vi "Add Tree Location.vi"(5 "Property Name":string, 7 "Property Value":string, 8 "error in (no error)":errorcluster, 9 "Tree Items Created In":variant, 10 "Tree Parent Tag In":string, 11 "TreeControl in":refnum<vi>) -> (0 "error out":errorcluster, 1 "Tree Items Created Out":variant, 2 "Tree Parent Tag Out":string)   [LabVIEW 2017, in "XTree.xctl"]
doc: "Adds a single tree location, if it does not already exist in the Tree Items Created variant."
uses:
  <vilib>/addons/_NIFileIO/XTree/XTree.xctl
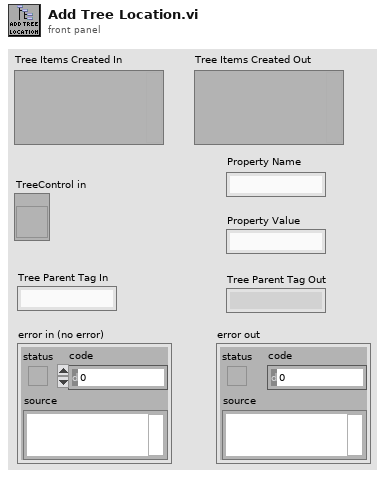
[diagram p1: front panel]
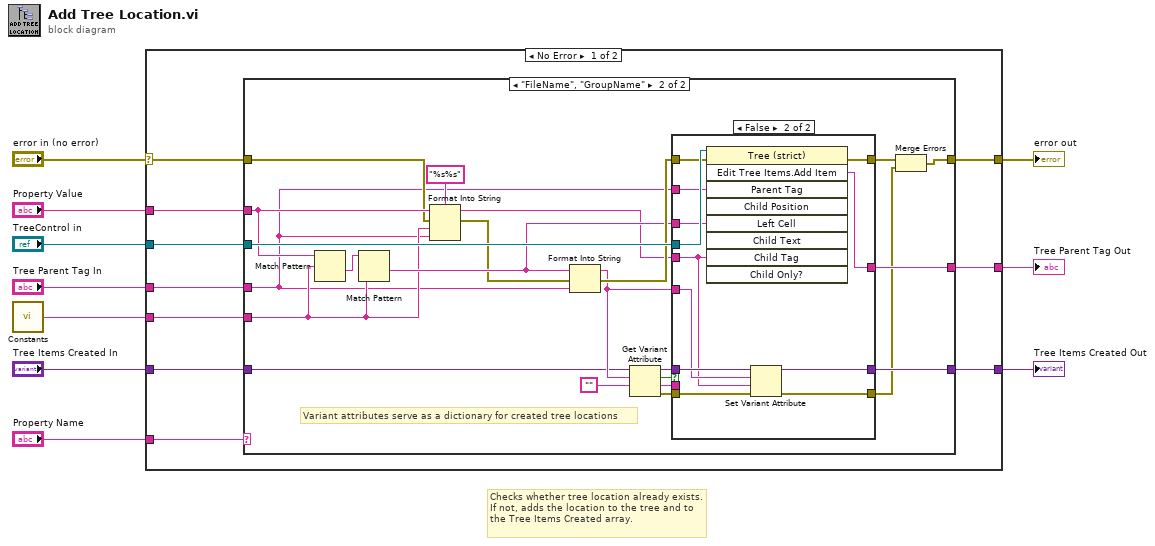
[diagram p0: block diagram]
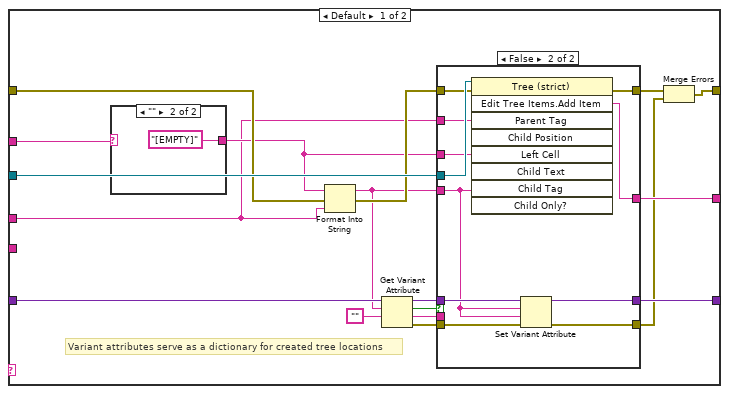
[diagram p2: hidden frame]
diagram:
  # "Checks whether tree location already exists. If not, adds the location to the tree and to the Tree Items Created array."
  n1 = call <vilib>:"Constants.vi"() -> ("String Delimeter"=w4:string)  [unwired: 5 in]
  n2 = case shown="No Error" "error in (no error)" {
    selector: "error in (no error)" -> [w17 w96]
    tunnel: "Tree Parent Tag In" -> [w15 w97]
    tunnel: [w20 w96] -> w9
    tunnel: [w19 w97] -> w8
    tunnel: "TreeControl in" -> [w18 _]
    tunnel: "Property Value" -> [w16 _]
    tunnel: w4 -> [w14 _]
    tunnel: "Property Name" -> [w13 _]
    tunnel: "Tree Items Created In" -> [w12 w95]
    tunnel: [w11 w95] -> w1
    frame No Error {
      n3 = case shown="\"FileName\", \"GroupName\"" w13 {
        tunnel: [w24 w58] -> w20
        tunnel: [w38 w78] -> w19
        tunnel: w18 -> [w37 w77]
        tunnel: w17 -> [w36 w72]
        tunnel: w16 -> [w35 w73]
        tunnel: w15 -> [w32 w67]
        tunnel: w14 -> [_ w70]
        tunnel: w12 -> [w31 w65]
        tunnel: [w26 w61] -> w11
        frame Default {
          # "Variant attributes serve as a dictionary for created tree locations"
          n4 = case shown="\"\"" w35 {
            selector: w35 -> [w39 _]
            tunnel: [w39 "[EMPTY]"] -> w33
            frame Default {
            }
            frame "" {
            }
          }
          n5 = Format Into String(initial string=w33, error in=w36, w32) -> (resulting string=w30:string, error out=w34:errorcluster)  [unwired: 1 in]
          n6 = Get Variant Attribute(Variant=w31, name=w30, default value (empty Variant)="") -> (duplicate Variant=w28:variant, found=w29:bool, value=w25:string, error out=w27:errorcluster)  [unwired: 1 in]
          n7 = case shown="False" w29 {
            tunnel: w37 -> [_ w55]
            tunnel: w34 -> [w44 w54]
            tunnel: [w43 w53] -> w38
            tunnel: [w44 w52] -> w23
            tunnel: w32 -> [_ w51]
            tunnel: w33 -> [_ w50]
            tunnel: w30 -> [_ w48]
            tunnel: w28 -> [w42 w49]
            tunnel: w27 -> [w41 w47]
            tunnel: [w42 w46] -> w26
            tunnel: w25 -> [w43 _]
            tunnel: [w41 w45] -> w22
            frame True {
            }
            frame False {
              n8 = invoke class="Tree (strict)" method="Edit Tree Items.Add Item"(reference=w55, error in=w54, "Parent Tag"=w51, "Left Cell"=w50, "Child Tag"=w48) -> (error out=w52:errorcluster, "Edit Tree Items:Add Item"=w53:string)  [unwired: 4 in, 7 out]
              n9 = Set Variant Attribute(Variant=w49, name=w48, value=w48, error in=w47) -> (Variant out=w46:variant, error out=w45:errorcluster)  [unwired: 1 out]
            }
          }
          n10 = Merge Errors(w23, w22) -> (w24:errorcluster)
        }
        frame "FileName", "GroupName" {
          # "Variant attributes serve as a dictionary for created tree locations"
          n11 = Match Pattern(string=w73, regular expression=w70) -> (after substring=w75:string)  [unwired: 1 in, 3 out]
          n12 = Match Pattern(string=w75, regular expression=w70) -> (after substring=w74:string)  [unwired: 1 in, 3 out]
          n13 = Format Into String(format string="%s%s", initial string=w73, error in=w72, w70, w67) -> (resulting string=w69:string, error out=w71:errorcluster)
          n14 = Format Into String(initial string=w74, error in=w71, w67) -> (resulting string=w66:string, error out=w76:errorcluster)  [unwired: 1 in]
          n15 = Get Variant Attribute(Variant=w65, name=w66, default value (empty Variant)="") -> (duplicate Variant=w63:variant, found=w64:bool, value=w60:string, error out=w62:errorcluster)  [unwired: 1 in]
          n16 = case shown="False" w64 {
            tunnel: w77 -> [_ w94]
            tunnel: w76 -> [w82 w93]
            tunnel: [w81 w92] -> w78
            tunnel: [w82 w91] -> w59
            tunnel: w67 -> [_ w90]
            tunnel: w66 -> [_ w86]
            tunnel: w69 -> [_ w85]
            tunnel: w74 -> [_ w89]
            tunnel: w63 -> [w80 w88]
            tunnel: w62 -> [w79 w87]
            tunnel: [w80 w84] -> w61
            tunnel: w60 -> [w81 _]
            tunnel: [w79 w83] -> w57
            frame True {
            }
            frame False {
              n17 = invoke class="Tree (strict)" method="Edit Tree Items.Add Item"(reference=w94, error in=w93, "Parent Tag"=w90, "Left Cell"=w89, "Child Tag"=w85) -> (error out=w91:errorcluster, "Edit Tree Items:Add Item"=w92:string)  [unwired: 4 in, 7 out]
              n18 = Set Variant Attribute(Variant=w88, name=w86, value=w85, error in=w87) -> (Variant out=w84:variant, error out=w83:errorcluster)  [unwired: 1 out]
            }
          }
          n19 = Merge Errors(w59, w57) -> (w58:errorcluster)
        }
      }
    }
    frame Error {
    }
  }
  "error out" <- w9
  "Tree Parent Tag Out" <- w8
  "Tree Items Created Out" <- w1
